vi "多定时器.vi"() -> ()   [LabVIEW 2011]
uses:
  Timer.lvclass
panel:
  out "Pulse":bool[](array[boolean])
  out "Time":bool[](array[boolean])
  out "经历时间":u32[](array[numeric])
  in  "stop":bool
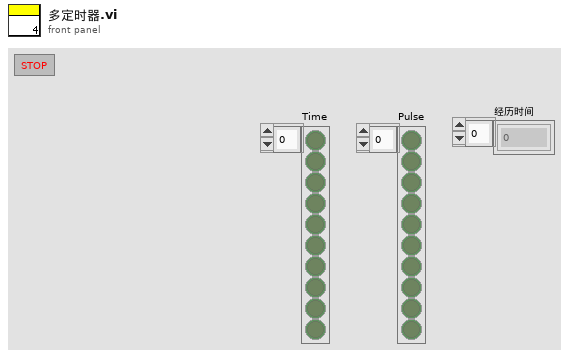
[diagram p1: front panel]
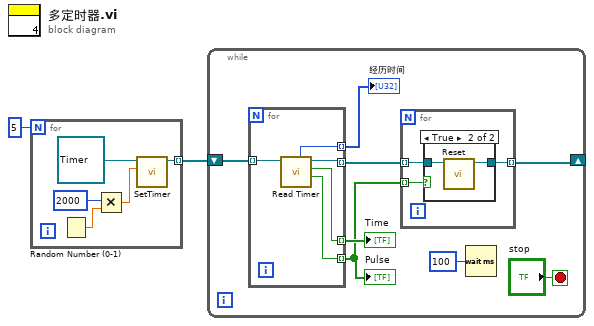
[diagram p0: block diagram]
diagram:
  n1 = for {
    N: 5 -> [_]
    tunnel: [w6] -> w1 mode=indexing
    n2 = Random Number (0-1)() -> (number: 0 to 1=w4:dbl)
    n3 = Multiply(x=u32 2000, y=w4) -> (x*y=w3:dbl)
    n4 = call "SetTimer.vi"("Set Timer"=w3, "Timer in"=refnum<class "Timer.lvclass"> refnum ("Timer.lvclass")) -> ("Timer out"=w6:refnum<class "Timer.lvclass">)  [unwired: 8 in, 1 out]
  }
  n5 = while {
    shift-right: [w11] -> _
    shift-left: w1 -> [w14]
    stop <- "stop" stop-if-true
    n6 = for {
      tunnel: w14 -> [w26] mode=indexing
      tunnel: [w25] -> w12 mode=indexing
      tunnel: [w24] -> w13 mode=indexing
      tunnel: [w23] -> w9 mode=indexing
      tunnel: [w22] -> w10 mode=indexing
      n7 = call "Read Timer.vi"("Timer in"=w26) -> ("Time?Pulse"=w23:bool, "Time?"=w22:bool, "Timer out"=w24:refnum<class "Timer.lvclass">, "Run"=w25:u32)  [unwired: 6 in, 1 out]
    }
    "经历时间" <- w12
    "Time" <- w10
    "Pulse" <- w9
    n8 = for {
      tunnel: w13 -> [w18] mode=indexing
      tunnel: [w17] -> w11 mode=indexing
      tunnel: w9 -> [w16] mode=indexing
      n9 = case shown="True" w16 {
        tunnel: [w19 w20] -> w17
        tunnel: w18 -> [w19 w21]
        frame False {
        }
        frame True {
          n10 = call "Reset.vi"("Timer in"=w21) -> ("Timer out"=w20:refnum<class "Timer.lvclass">)  [unwired: 9 in, 1 out]
        }
      }
    }
    n11 = Wait (ms)(milliseconds to wait=u32 100) -> ()  [unwired: 1 out]
  }
